vi "ReportHead.vi"(8 "error in (no error)":errorcluster caption="错误输入（无错误）", 11 "产品状态":string) -> (0 "error out":errorcluster caption="错误输出", 3 "report out":refnum<class "NI_report.lvclass"> caption="报表输出")   [LabVIEW 2020]
uses:
  <vilib>/Utility/NIReport.llb/NI_report.lvclass
  <vilib>/addons/_office/_exclsub.llb/font.ctl
  Database/Global1.vi
  Global_Variable/Global.vi
  <vilib>/addons/_office/NI_ReportGenerationToolkit.lvlib
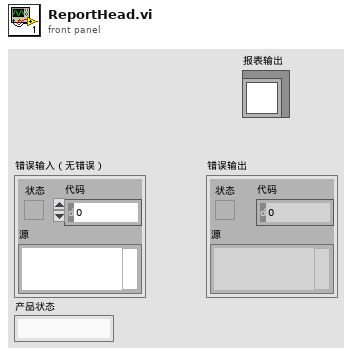
[diagram p1: front panel]
types:
  T1 = cluster{"操作者编号":string, "操作者姓名":string, "操作者权限":string, "联机状态":string, "产品型号":string, "产品状态":string}
  T2 = cluster{"top":dbl, "left":dbl, "right":dbl, "bottom":dbl}
  T3 = cluster{"Charset (-1)":i16, "Weight (-1)":i16, "Name":string, "Size":string}
  T4 = cluster{"Italic":enum16{"Italic Unchanged", "Italic On", "Italic Off"}, "Strike Through":enum16{"Strike Through Unchanged", "Strike Through On", "Strike Through Off"}, "Underline":enum16{"Underline Unchanged", "Underline On", "Underline Off"}, "Bold":enum16{"Bold Unchanged", "Bold On", "Bold Off"}}
  T5 = typedef "NI_ReportGenerationToolkit.lvlib/font.ctl" = cluster{"font name":string, "font size":dbl, "bold":u16, "italic":u16, "underline":u16, "strike through":u16, "font color":u32}
  T6 = enum16{"maximized", "minimized", "normal", "no change"}
  T7 = enum16{"Standard Report", "HTML", "Word", "Excel"}
  T8 = cluster{"用户编号":string, "用户名":string, "用户密码(密文)":string, "用户权限":string}
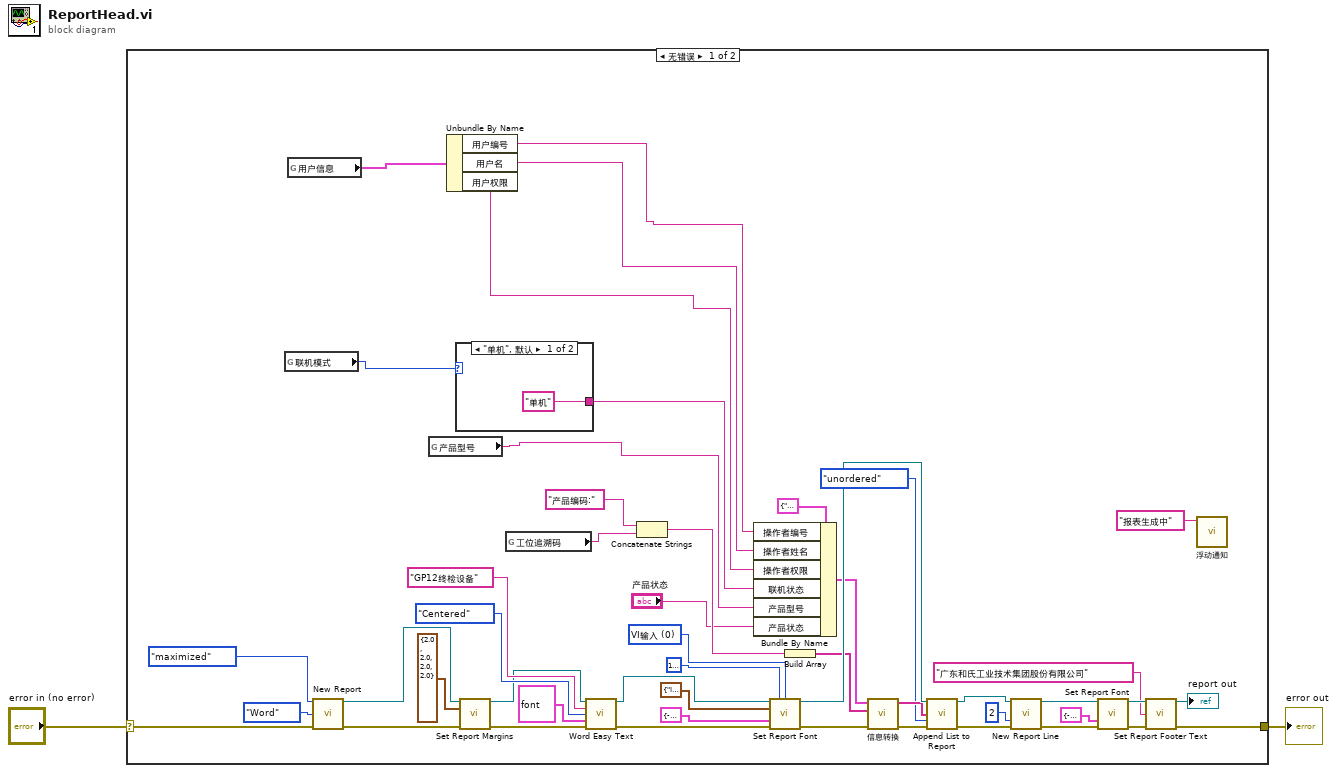
[diagram p0: block diagram]
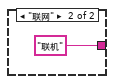
[diagram p2: hidden frame]
diagram:
  n1 = case shown="无错误" "error in (no error)" {
    selector: "error in (no error)" -> [w23 w53]
    tunnel: [w19 w53] -> w1
    frame No Error {
      w43 = u16 0 items=["VI输入", "字体对话框"] ("font settings source")
      n2 = global read "Global1.vi" "联机模式"() -> (w5:enum16{"单机", "联网"})
      n3 = global read "Global1.vi" "用户信息"() -> (w6:T8)
      n4 = call <vilib>:"New Report.vi"("window state (normal)"=T6."maximized", "report type"=T7."Word", "error in (no error)"=w23) -> ("report out"=w36:refnum<class "NI_report.lvclass">, "error out"=w33:errorcluster)  [unwired: 11 in]
      n5 = global read "Global.vi" "产品型号"() -> (w4:string)
      n6 = Unbundle By Name(w6) -> ("用户编号"=w9:string, "用户名"=w8:string, "用户权限"=w7:string)
      n7 = case shown="\"单机\", 默认" w5 {
        tunnel: ["单机" "联机"] -> w17
        frame "单机", Default {
        }
        frame "联网" {
        }
      }
      n8 = call-dynamic "Set Report Margins.vi"("report in"=w36, "margins (1.00)"=T2 {"top"=2.0, "left"=2.0, "right"=2.0, "bottom"=2.0}, "error in (no error)"=w33) -> ("report out"=w35:refnum<class "NI_report.lvclass">, "error out"=w34:errorcluster)  [unwired: 10 in, 1 out]
      n9 = global read "Global1.vi" "工位追溯码"() -> (w3:string)
      n10 = call <vilib>:"Word Easy Text.vi"("report in"=w35, "text"="GP12终检设备", "alignment (left)"=enum16{"Left", "Centered", "Right", "Justify"}."Centered", "font"=T5 {"font name"="楷体", "font size"=26.0, "bold"=1, "italic"=2, "underline"=2, "strike through"=2, "font color"=16777228}, "error in (no error)"=w34) -> ("report out"=w45:refnum<class "NI_report.lvclass">, "error out"=w44:errorcluster)  [unwired: 8 in, 1 out]
      n11 = Concatenate Strings("产品编码:", w3) -> (w13:string)
      n12 = Bundle By Name(cluster=T1 {"操作者编号"="001", "操作者姓名"="Administrator", "操作者权限"="系统管理员", "联机状态"="单机", "产品型号"="SL7202", "产品状态"=""} ("测试信息"), "操作者编号"=w9, "操作者姓名"=w8, "操作者权限"=w7, "联机状态"=w17, "产品型号"=w4, "产品状态"="产品状态") -> (w15:T1)
      n13 = call-dynamic "Set Report Font.vi"("report in"=w45, "text color (unchanged)"=u32 16777224, "font settings source (VI Inputs)"=w43, "text options"=T4 {"Italic"=enum."Italic Off", "Strike Through"=enum."Strike Through Unchanged", "Underline"=enum."Underline Off", "Bold"=enum."Bold Off"}, "font settings"=T3 {"Charset (-1)"=-1, "Weight (-1)"=-1, "Name"="微软雅黑 Light", "Size"="12 "}, "error in (no error)"=w44) -> ("report out"=w31:refnum<class "NI_report.lvclass">, "error out"=w22:errorcluster)  [unwired: 7 in, 1 out]
      n14 = Build Array(w13) -> (w12:string[])
      n15 = call "信息转换.vi"("错误输入（无错误）"=w22, "追溯码"=w12, "测试信息"=w15) -> ("错误输出"=w21:errorcluster, "信息输出"=w24:string[])  [unwired: 7 in]
      n16 = call-dynamic "Append List to Report.vi"("report in"=w31, "list elements"=w24, "list type (ordered)"=enum16{"unordered", "ordered"}."unordered", "error in (no error)"=w21) -> ("report out"=w26:refnum<class "NI_report.lvclass">, "error out"=w25:errorcluster)  [unwired: 8 in, 2 out]
      n17 = call-dynamic "New Report Line.vi"("report in"=w26, "number of lines (1)"=2, "error in (no error)"=w25) -> ("report out"=w29:refnum<class "NI_report.lvclass">, "error out"=w30:errorcluster)  [unwired: 11 in]
      n18 = call-dynamic "Set Report Font.vi"("report in"=w29, "font settings"=T3 {"Charset (-1)"=-1, "Weight (-1)"=-1, "Name"="楷体", "Size"="9 "}, "error in (no error)"=w30) -> ("report out"=w40:refnum<class "NI_report.lvclass">, "error out"=w39:errorcluster)  [unwired: 10 in, 1 out]
      n19 = call-dynamic "Set Report Footer Text.vi"("report in"=w40, "center footer text"="广东和氏工业技术集团股份有限公司", "error in (no error)"=w39) -> ("report out"=→"report out":refnum<class "NI_report.lvclass">, "error out"=w19:errorcluster)  [unwired: 11 in]
      n20 = call "浮动通知.vi"("通知内容"="报表生成中" ("Status")) -> ()  [unwired: 11 in]
    }
    frame Error {
    }
  }
  "error out" <- w1
